vi "Exercice3.vi"() -> ()   [LabVIEW 2018]
panel:
  out "Led":bool
  out "Prénom":string
  out "Nom":string
  in  "Nom brut":string
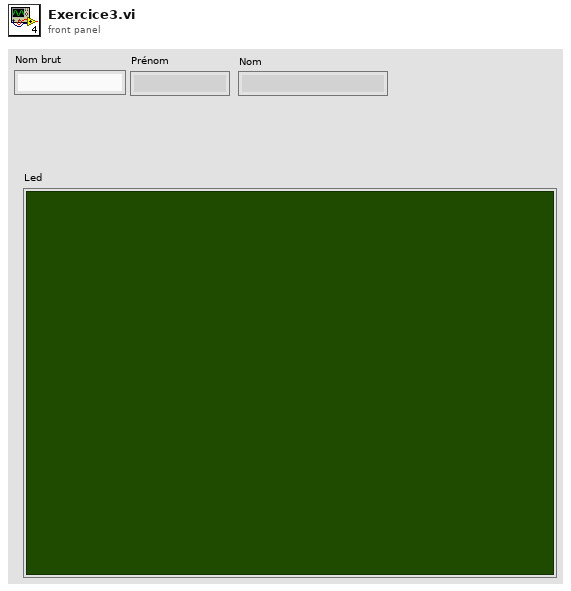
[diagram p1: front panel]
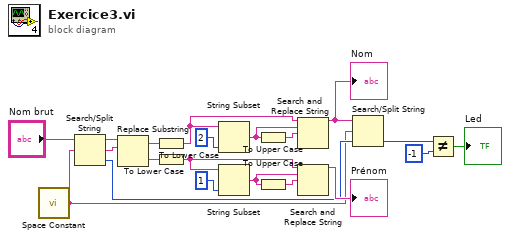
[diagram p0: block diagram]
diagram:
  n1 = call <vilib>:"Space Constant.vi"() -> ("String"=w5:string)
  n2 = Search/Split String(string="Nom brut", search string/char (-)=w5) -> (substring before match=w12:string, match + rest of string=w11:string, offset of match=w6:i32)  [unwired: 1 in]
  n3 = Replace Substring(4:w11, 5:w12) -> (0:w9:string, 1:w10:string)  [unwired: 2 in]
  n4 = To Lower Case(string=w10) -> (all lower case string=w20:string)
  n5 = To Lower Case(string=w9) -> (all lower case string=w13:string)
  n6 = String Subset(string=w20, length (rest)=2 ("length (rest)")) -> (substring=w18:string)  [unwired: 1 in]
  n7 = String Subset(string=w13, length (rest)=1 ("length (rest)")) -> (substring=w15:string)  [unwired: 1 in]
  n8 = To Upper Case(1:w18) -> (0:w17:string)
  n9 = To Upper Case(1:w15) -> (0:w14:string)
  n10 = Search and Replace String(input string=w20, search string=w18, replace string=w17) -> (result string=w4:string)  [unwired: 5 in, 3 out]
  "Nom" <- w4
  n11 = Search and Replace String(input string=w13, search string=w15, replace string=w14) -> (result string=→"Prénom":string)  [unwired: 5 in, 3 out]
  n12 = Search/Split String(string=w4, search string/char (-)=w5, offset (0)=w6) -> (offset of match=w3:i32)  [unwired: 2 out]
  n13 = Not Equal?(x=w3, y=-1) -> (x != y?=→"Led":bool)
